vi "final_tack_builder.vi"(6 "Distance for tack to travel (m)":dbl, 7 "Amount to extend tack waypoints (m)":dbl, 8 "Angle (Other leyline -> WP) (deg)":dbl, 9 "Angle (Final leyline -> WP) (deg)":dbl, 10 "Other leyline (deg)":dbl, 11 "Proposed WP array IN":refnum<class "Waypoint.lvclass">[](array[class])) -> (3 "Proposed WP array":refnum<class "Waypoint.lvclass">[](array[class]))   [LabVIEW 2013]
doc: "This VI takes the information to build the last tack of a series and adds that point to a created array.\n\nEric Schneider, September 2014"
uses:
  Classes/Waypoint/Waypoint.lvclass
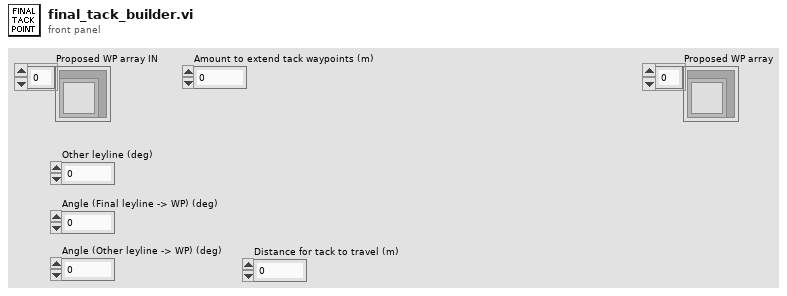
[diagram p1: front panel]
types:
  T1 = typedef "UTM Location.ctl" = cluster{"UTM Zone":dbl, "Hemisphere":enum16{"North", "South"}, "East":dbl, "North":dbl}
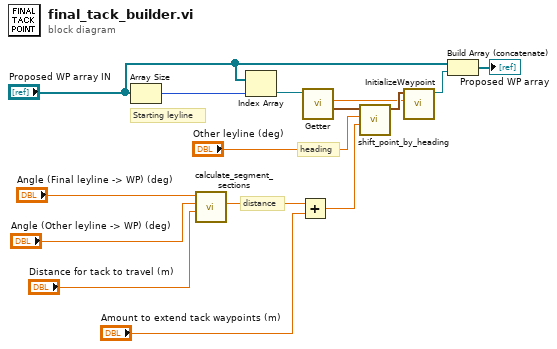
[diagram p0: block diagram]
diagram:
  # "distance"
  # "heading"
  # "Starting leyline"
  n1 = Array Size(array="Proposed WP array IN") -> (size(s)=w5:i32)
  n2 = call "calculate_segment_sections.vi"("range (m)"="Distance for tack to travel (m)", "Angle WP to second leyline (deg)"="Angle (Other leyline -> WP) (deg)", "Angle WP to first leyline (deg)"="Angle (Final leyline -> WP) (deg)") -> ("Length of second leg (m)"=w7:dbl)  [unwired: 5 in, 3 out]
  n3 = Index Array(array="Proposed WP array IN", index=w5) -> (element=w3:refnum<class "Waypoint.lvclass">)
  n4 = Add(x=w7, y="Amount to extend tack waypoints (m)") -> (x+y=w9:dbl)
  n5 = call "Getter.vi"("Waypoint In"=w3) -> ("Coords"=w1:T1, "Tolerance (meters?)"=w2:dbl)  [unwired: 6 in, 3 out]
  n6 = call "shift_point_by_heading.vi"("Distance (m)"=w9, "Heading (deg)"="Other leyline (deg)", "UTM Point"=w1) -> ("Shifted UTM Point"=w11:T1)  [unwired: 8 in]
  n7 = call "InitializeWaypoint.vi"("Tolerance (meters?) (0)"=w2, "Coords"=w11) -> ("Waypoint Out"=w10:refnum<class "Waypoint.lvclass">)  [unwired: 9 in]
  n8 = Build Array (concatenate)("Proposed WP array IN", w10) -> (→"Proposed WP array":refnum<class "Waypoint.lvclass">[])
